vi "MC5e Unit Editor.vi"(6 "Mode":T2, 8 "error in":errorcluster, 11 "index":i32) -> (0 "error out":errorcluster, 2 "Cancelled":bool)   [LabVIEW 2020]
uses:
  MC5e Editor modes.ctl
  MC5e Unit Header.ctl
  MC5e Unit.ctl
  MC5e Terrain types.ctl
  MC5e Squad_Info.ctl
  MC5e Size_Categories.ctl
  Location.ctl
  MC5e Unit_Manager_Modes.ctl
panel:
  in  "Unit Info":T1
  in  "OK Button":bool
  in  "Cancel Button":bool
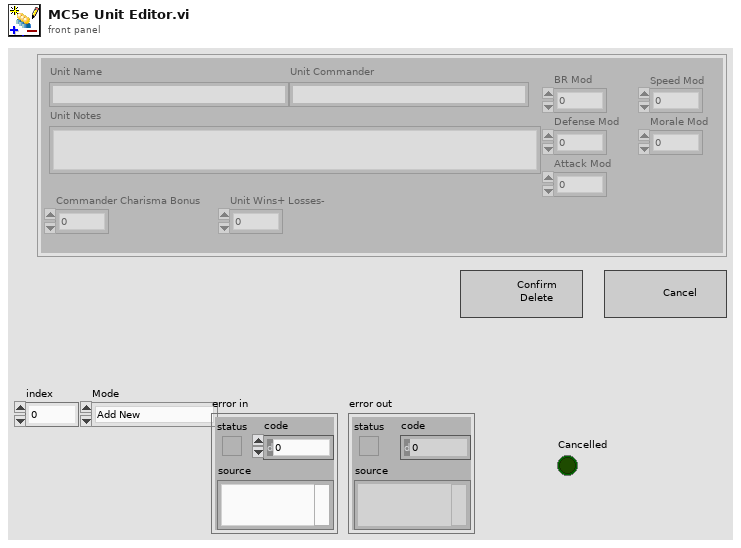
[diagram p1: front panel]
types:
  T1 = typedef "MC5e Unit Header.ctl" = cluster{"Unit Name":string, "Unit Commander":string, "Morale Mod":i32, "BR Mod":i32, "Defense Mod":i32, "Speed Mod":i32, "Unit Notes":string, "Attack Mod":i32, "Unit Wins+ Losses-":i32, "Commander Charisma Bonus":i32}
  T2 = typedef "MC5e Editor modes.ctl" = enum16{"Add New", "Copy Selected", "Delete Selected", "Edit Selected"}
  T3 = typedef "MC5e Unit.ctl" = cluster{"Unit Fatigue Level":enum16{"Not Fatigued", "Fatigued", "Seriously Fatigued"}, "Flying Unit":bool, "Mounted Unit":bool, "Defending from Stronghold":bool, "Difficult Terrain Types":T4, "Squads in Unit":T5[], "Unit Info":T1, "Range":i32, "BR":i32, "Speed":i32, "Morale":i32, "Current BR":i32, "Location":T7, "Capacity %":i32}
  T4 = typedef "MC5e Terrain types.ctl" = i32[]
  T5 = typedef "MC5e Squad_Info.ctl" = cluster{"Squad Name":string, "# Soldiers":u16, "Battle Rating":u16, "Flying":bool, "Mounted":bool, "Speed":u16, "Range":u16, "Morale":i32, "Max Endurance":u16, "Current Endurance":i32, "Size":T6, "Space Taken":u16, "Difficult Terrain":i32[], "CR":u16, "Special / Notes":string}
  T6 = typedef "MC5e Size_Categories.ctl" = enum16{"Tiny", "Small", "Medium", "Large", "Huge", "Gargantuan"}
  T7 = typedef "Location.ctl" = cluster{"X coordinate":dbl, "Y coordinate":dbl}
  T8 = enum8{"Enabled", "Disabled", "Disabled and Grayed Out"}
  T9 = typedef "MC5e Unit_Manager_Modes.ctl" = enum16{"Initialize", "Add Unit", "Delete Unit", "Get Unit", "Load Set", "Replace Unit"}
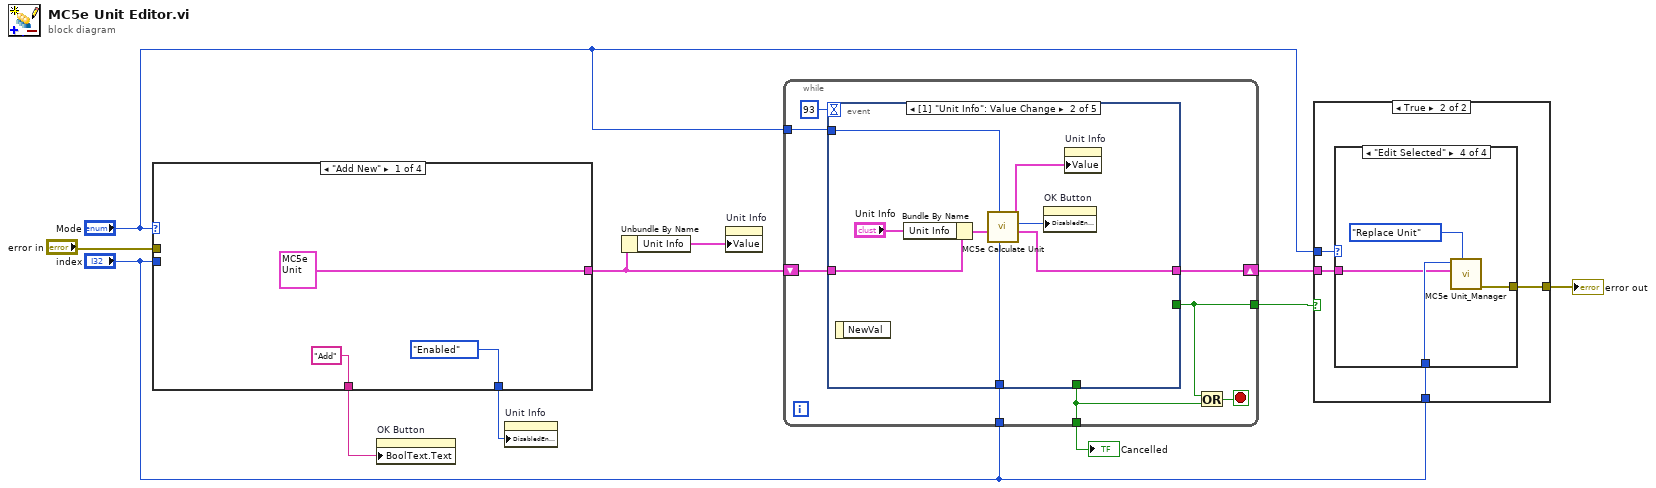
[diagram p0: block diagram]
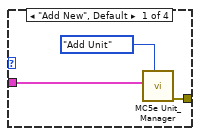
[diagram p3: hidden frame]
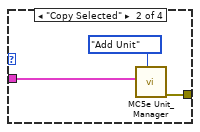
[diagram p4: hidden frame]
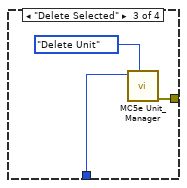
[diagram p5: hidden frame]
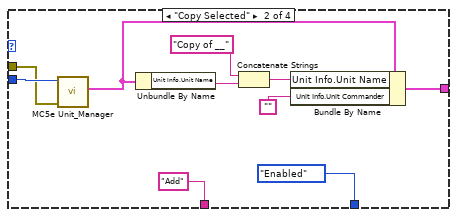
[diagram p6: hidden frame]
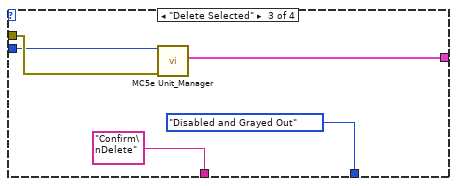
[diagram p7: hidden frame]
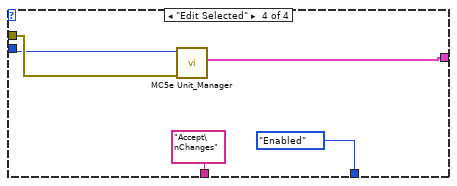
[diagram p8: hidden frame]
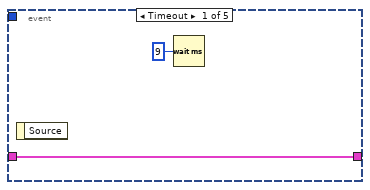
[diagram p9: hidden frame]
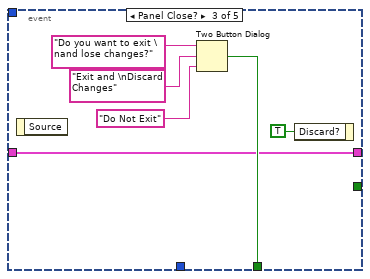
[diagram p10: hidden frame]
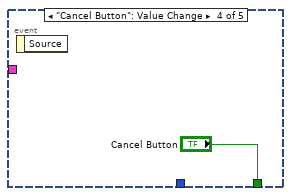
[diagram p11: hidden frame]
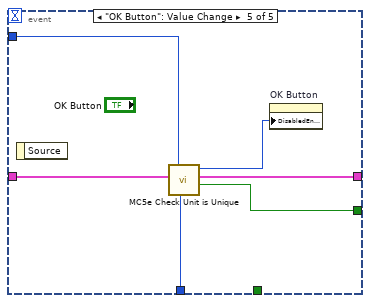
[diagram p12: hidden frame]
diagram:
  n1 = case shown="\"Add New\"" "Mode" {
    tunnel: "index" -> [_ w20 w27 w32]
    tunnel: ["Add" ("Caption.Text") "Add" ("Caption.Text") "Confirm\nDelete" ("Caption.Text") "Accept\nChanges" ("Caption.Text")] -> w11
    tunnel: "error in" -> [_ w19 w28 w33]
    tunnel: [T8."Enabled" ("Disabled") T8."Enabled" ("Disabled") T8."Disabled and Grayed Out" ("Disabled") T8."Enabled" ("Disabled")] -> w4
    tunnel: [T3 {"Unit Fatigue Level"=enum."Not Fatigued", "Flying Unit"=FALSE, "Mounted Unit"=FALSE, "Defending from Stronghold"=FALSE, "Difficult Terrain Types"=[0, 1, 3, 6, 7], "Squads in Unit"=[], "Unit Info"={"Unit Name"="", "Unit Commander"="", "Morale Mod"=0, "BR Mod"=0, "Defense Mod"=0, "Speed Mod"=0, "Unit Notes"="", "Attack Mod"=0, "Unit Wins+ Losses-"=0, "Commander Charisma Bonus"=0}, "Range"=0, "BR"=0, "Speed"=0, "Morale"=0, "Current BR"=0, "Location"={"X coordinate"=0.0, "Y coordinate"=0.0}, "Capacity %"=0} ("Unit") w15 w25 w30] -> w2
    frame "Add New" {
    }
    frame "Copy Selected" {
      n2 = call "MC5e Unit_Manager.vi"("error in"=w19, "index (get/delete/replace)"=w20) -> ("Unit"=w18:T3)  [unwired: 6 in, 3 out]
      n3 = Unbundle By Name(w18) -> ("Unit Info.Unit Name"=w24:string)
      n4 = Concatenate Strings("Copy of __" ("string"), w24) -> (w21:string)
      n5 = Bundle By Name(cluster=w18, "Unit Info.Unit Name"=w21, "Unit Info.Unit Commander"="") -> (w15:T3)
    }
    frame "Delete Selected" {
      n6 = call "MC5e Unit_Manager.vi"("error in"=w28, "index (get/delete/replace)"=w27) -> ("Unit"=w25:T3)  [unwired: 6 in, 3 out]
    }
    frame "Edit Selected" {
      n7 = call "MC5e Unit_Manager.vi"("error in"=w33, "index (get/delete/replace)"=w32) -> ("Unit"=w30:T3)  [unwired: 6 in, 3 out]
    }
  }
  n8 = property on="OK Button" class="Bool"("BoolText.Text"=w11) -> ()  [unwired: 2 in, 2 out]
  n9 = property on="Unit Info" class="Clust (strict)"("DisabledEnum"=w4) -> ()  [unwired: 2 in, 2 out]
  n10 = Unbundle By Name(w2) -> ("Unit Info"=w1:T1)
  n11 = property on="Unit Info" class="Clust (strict)"("Value"=w1) -> ()  [unwired: 2 in, 2 out]
  n12 = while {
    tunnel: [w39] -> w10
    tunnel: [w41] -> w7
    tunnel: "Mode" -> [w38]
    tunnel: "index" -> [w37]
    shift-right: [w35] -> w3
    shift-left: w2 -> [w36]
    stop <- w40 stop-if-true
    n13 = event shown="[1] \"Unit Info\": Value Change" {
      selector: _ -> [_ _ _ _ _]
      dyn-events: _ -> [_ _ _ _ _]
      timeout: 93 -> [_ _ _ _ _]
      tunnel: [_ _ w54 "Cancel Button" _] -> w41
      tunnel: [_ _ _ _ w62] -> w39
      tunnel: w38 -> [_ w52 _ _ w60]
      tunnel: w37 -> [_ w50 _ _ w63]
      tunnel: w36 -> [w43 w47 w53 _ w64]
      tunnel: [w43 w49 w53 _ w61] -> w35
      event Timeout {
        n14 = event-data() -> ()  [unwired: 1 in, 1 out]
        n15 = Wait (ms)(milliseconds to wait=u32 9) -> ()  [unwired: 1 out]
      }
      event Value Change {
        n16 = event-data() -> ()  [unwired: 1 in, 1 out]
        n17 = Bundle By Name(cluster=w47, "Unit Info"="Unit Info") -> (w45:T3)
        n18 = call "MC5e Calculate Unit.vi"("index"=w50, "Mode"=w52, "Unit In"=w45) -> ("Unit Out"=w49:T3, "OK Button Disabled?"=w51:T8, "Unit Info Out"=w48:T1)  [unwired: 6 in]
        n19 = property on="OK Button" class="Bool"("DisabledEnum"=w51) -> ()  [unwired: 2 in, 2 out]
        n20 = property on="Unit Info" class="Clust (strict)"("Value"=w48) -> ()  [unwired: 2 in, 2 out]
      }
      event Panel Close? {
        n21 = event-data() -> ()  [unwired: 1 in, 1 out]
        n22 = Two Button Dialog(message="Do you want to exit \nand lose changes?", 1:"Do Not Exit" ("F button name (\"Cancel\")"), 2:"Exit and \nDiscard Changes" ("T button name (\"OK\")")) -> (T button?=w54:bool)
        n23 = event-data("Discard?"=TRUE) -> ()  [unwired: 1 in, 1 out]
      }
      event "Cancel Button": Value Change {
        n24 = event-data() -> ()  [unwired: 1 in, 1 out]
      }
      event "OK Button": Value Change {
        n25 = event-data() -> ()  [unwired: 1 in, 1 out]
        n26 = call "MC5e Check Unit is Unique.vi"("index"=w63, "Mode"=w60, "Unit"=w64) -> ("Unit Name is Valid"=w62:bool, "Unit Out (Duplicate)"=w61:T3, "OK Button Disabled?"=w65:T8)  [unwired: 6 in]
        n27 = property on="OK Button" class="Bool"("DisabledEnum"=w65) -> ()  [unwired: 2 in, 2 out]
      }
    }
    n28 = Or(x=w39, y=w41) -> (x .or. y?=w40:bool)
  }
  "Cancelled" <- w7
  n29 = case shown="True" w10 {
    tunnel: "Mode" -> [_ w69]
    tunnel: "index" -> [_ w68]
    tunnel: [_ w67] -> w9
    tunnel: w3 -> [_ w66]
    frame False {
    }
    frame True {
      n30 = case shown="\"Edit Selected\"" w69 {
        tunnel: w68 -> [_ _ w77 w80]
        tunnel: [w70 w74 w76 w81] -> w67
        tunnel: w66 -> [w71 w73 _ w79]
        frame "Add New", Default {
          n31 = call "MC5e Unit_Manager.vi"("Mode (Get)"=MC5e_Unit_Manager_Modes."Add Unit", "Unit In (Add/Replace)"=w71) -> ("error out"=w70:errorcluster)  [unwired: 6 in, 3 out]
        }
        frame "Copy Selected" {
          n32 = call "MC5e Unit_Manager.vi"("Mode (Get)"=MC5e_Unit_Manager_Modes."Add Unit", "Unit In (Add/Replace)"=w73) -> ("error out"=w74:errorcluster)  [unwired: 6 in, 3 out]
        }
        frame "Delete Selected" {
          n33 = call "MC5e Unit_Manager.vi"("Mode (Get)"=MC5e_Unit_Manager_Modes."Delete Unit", "index (get/delete/replace)"=w77) -> ("error out"=w76:errorcluster)  [unwired: 6 in, 3 out]
        }
        frame "Edit Selected" {
          n34 = call "MC5e Unit_Manager.vi"("Mode (Get)"=MC5e_Unit_Manager_Modes."Replace Unit", "Unit In (Add/Replace)"=w79, "index (get/delete/replace)"=w80) -> ("error out"=w81:errorcluster)  [unwired: 5 in, 3 out]
        }
      }
    }
  }
  "error out" <- w9
